vi "15_LLAMADA_DINÁMICA_COVIF_19.vi"() -> ()   [LabVIEW 2019]
panel:
  out "OUT":dbl
  out "error out":errorcluster
  in  "A":dbl
  in  "B":dbl
  in  "C":dbl
  in  "error in":errorcluster
  in  "vi path":path
  in  "type specifier VI Refnum (for type only)":refnum<vi>
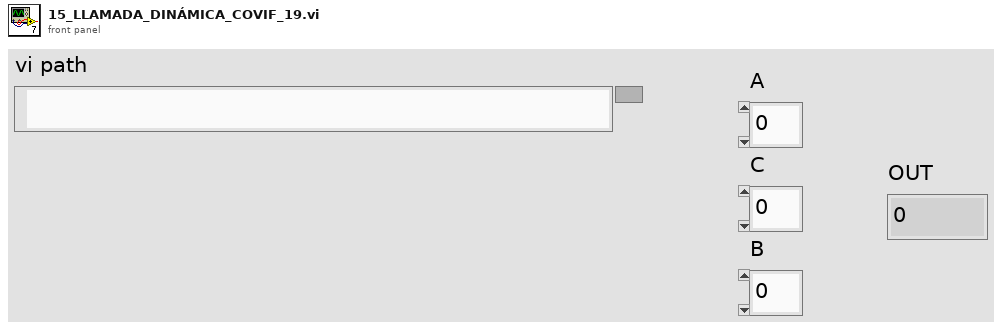
[diagram p1: front panel]
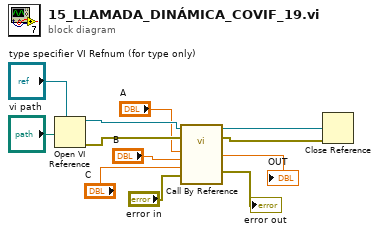
[diagram p0: block diagram]
diagram:
  n1 = Open VI Reference(type specifier VI Refnum (for type only)="type specifier VI Refnum (for type only)", vi path="vi path") -> (vi reference=w10:refnum<vi>, error out=w9:errorcluster)  [unwired: 4 in]
  n2 = call-by-ref "?"(reference=w10, error in=w9, "error in"="error in", "C"="C", "B"="B", "A"="A") -> (reference out=w8:refnum<vi>, error out=w7:errorcluster, 0:"error out"=→"error out":errorcluster, "OUT"=→"OUT":dbl)
  n3 = Close Reference(reference=w8, error in (no error)=w7) -> ()  [unwired: 1 out]
